vi "demo_Nigel AI Advisor.vi"(11 "Stop Demo":refnum<user-event>) -> ()   [LabVIEW 2020]
panel:
  # "LabVIEW 2025 Q3 - Nigel AI Advisor\n\nIncrease your productivity with the help of an experienced test and measured advisor. \nGet programming advice, learn LabVIEW concepts, and more!\nRequires an active subscription or SSP with LabVIEW Professional Edition\n\nLearn more at https://www.ni.com/en/shop/software-portfolio/nigel.html."
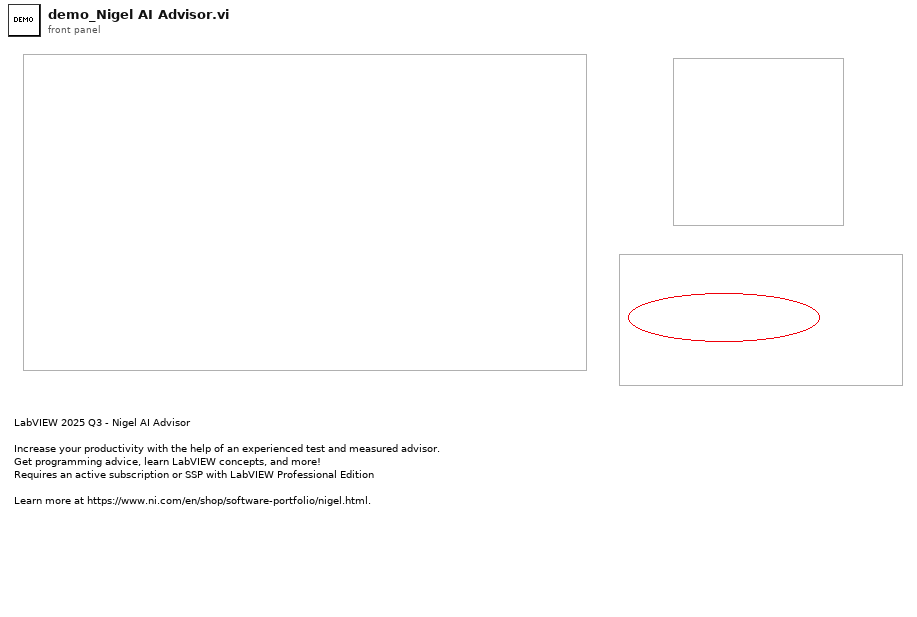
[diagram p1: front panel]
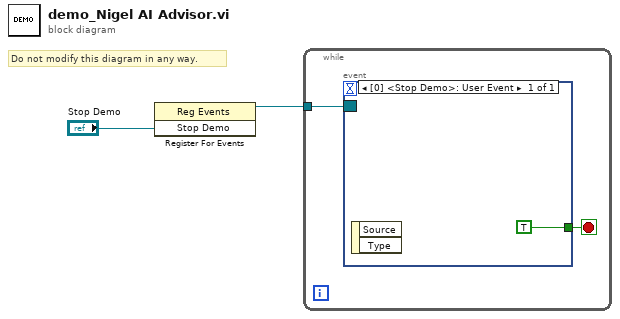
[diagram p0: block diagram]
diagram:
  # "Do not modify this diagram in any way."
  n1 = register-events("Stop Demo") -> (reference out=w1:refnum<event-registration>)  [unwired: 2 in, 1 out]
  n2 = while {
    tunnel: w1 -> [w4]
    stop <- w3 stop-if-true
    n3 = event shown="[0] <Stop Demo>: User Event" {
      selector: w4 -> [_]
      dyn-events: _ -> [_]
      timeout: _ -> [_]
      tunnel: [TRUE] -> w3
      event User Event {
        n4 = event-data() -> ()  [unwired: 1 in, 2 out]
      }
    }
  }
